vi "F6_1.vi"(8 "error in (no error)":errorcluster, 9 "data":u8[](array[numeric]), 10 "function":u8, 11 "device data model in":refnum<class "Standard Data Model1.lvclass">) -> (0 "error out":errorcluster, 1 "data return":u8[](array[numeric]), 2 "function return":u8, 3 "device data model out":refnum<class "Standard Data Model1.lvclass">)   [LabVIEW 2021, in "NI_modbus_upd.lvlib" / "Standard Data Model1.lvclass"]
doc: "Executes function code 6"
uses:
  Standard Data Model1.lvclass
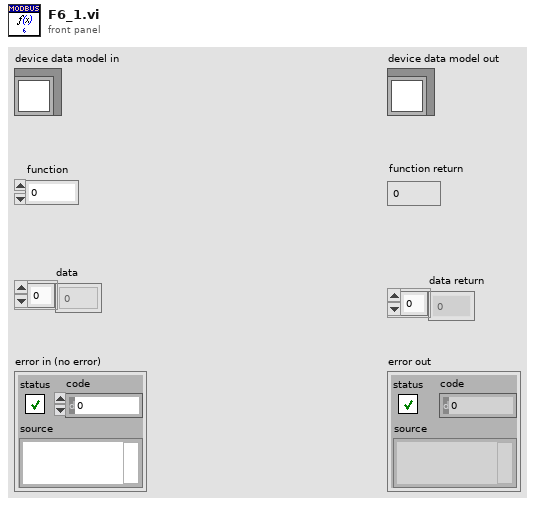
[diagram p1: front panel]
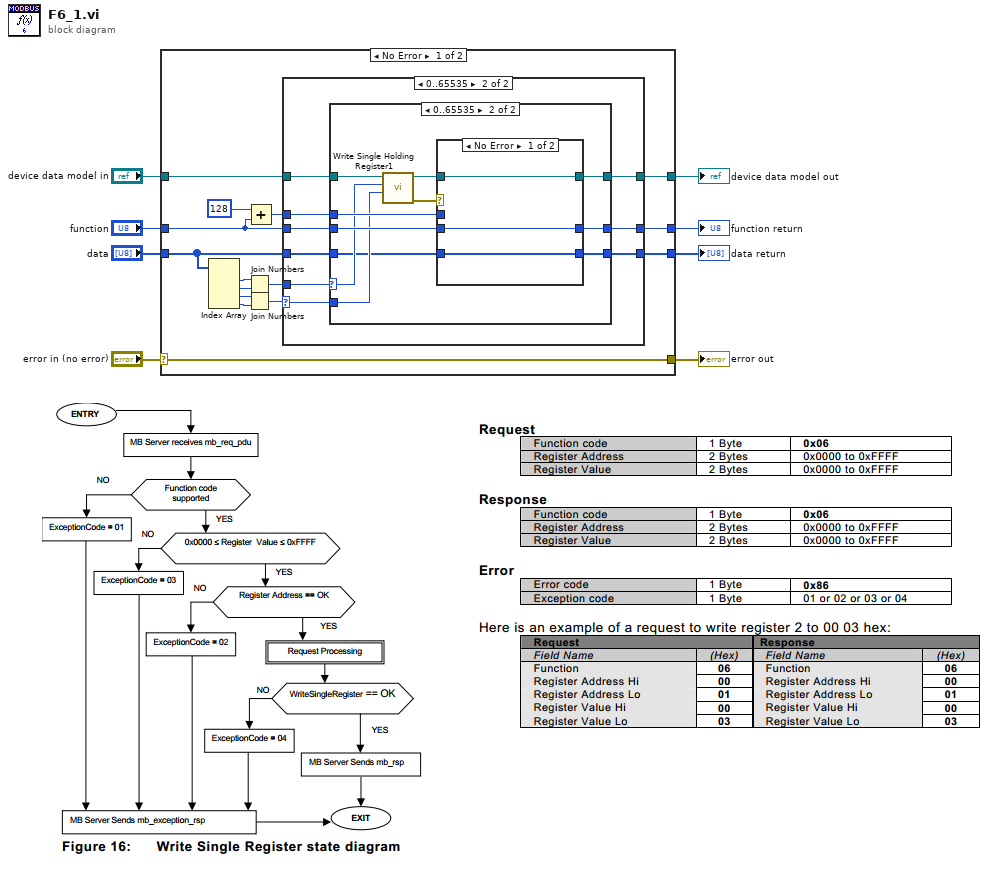
[diagram p0: block diagram]
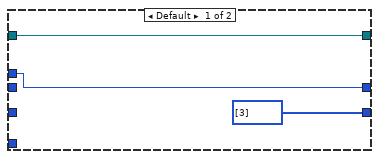
[diagram p2: hidden frame]
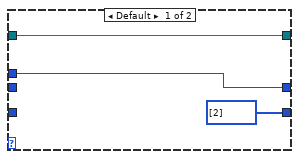
[diagram p3: hidden frame]
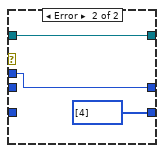
[diagram p4: hidden frame]
diagram:
  n1 = case shown="No Error" "error in (no error)" {
    selector: "error in (no error)" -> [w23 w59]
    tunnel: [w23 w59] -> w7
    tunnel: [w17 w58] -> w5
    tunnel: "device data model in" -> [w16 w58]
    tunnel: "function" -> [w13 w57]
    tunnel: "data" -> [w9 w56]
    tunnel: [w12 w57] -> w2
    tunnel: [w11 w56] -> w1
    frame No Error {
      n2 = Index Array(array=w9) -> (element #1=w21:u8, element #2=w22:u8, element #3=w20:u8, element #4=w19:u8)  [unwired: 4 in]
      n3 = Join Numbers(hi=w21, lo=w22) -> ((hi.lo)=w10:u16)
      n4 = Join Numbers(hi=w20, lo=w19) -> ((hi.lo)=w18:u16)
      n5 = Add(x=u8 128, y=w13) -> (x+y=w14:u8)
      n6 = case shown="0..65535" w18 {
        selector: w18 -> [_ w35]
        tunnel: [w26 w34] -> w17
        tunnel: w16 -> [w26 w33]
        tunnel: w14 -> [w25 w32]
        tunnel: w13 -> [_ w30]
        tunnel: [w25 w31] -> w12
        tunnel: [u8[] [3] ("Data Return") w29] -> w11
        tunnel: w10 -> [_ w28]
        tunnel: w9 -> [_ w27]
        frame Default {
        }
        frame 0..65535 {
          n7 = case shown="0..65535" w28 {
            selector: w28 -> [_ w42]
            tunnel: w35 -> [_ w43]
            tunnel: [w38 w49] -> w34
            tunnel: w33 -> [w38 w41]
            tunnel: w32 -> [w37 w48]
            tunnel: [w37 w46] -> w31
            tunnel: w30 -> [_ w47]
            tunnel: [u8[] [2] ("Data Return") w45] -> w29
            tunnel: w27 -> [_ w39]
            frame Default {
            }
            frame 0..65535 {
              n8 = call "Write Single Holding Register1.vi"("register value"=w43, "address"=w42, "device data model in"=w41) -> ("error out"=w40:errorcluster, "device data model out"=w44:refnum<class "Standard Data Model1.lvclass">)  [unwired: 7 in]
              n9 = case shown="No Error" w40 {
                tunnel: w44 -> [w52 w55]
                tunnel: [w52 w55] -> w49
                tunnel: w48 -> [_ w54]
                tunnel: w47 -> [w51 _]
                tunnel: [w51 w54] -> w46
                tunnel: [w50 u8[] [4]] -> w45
                tunnel: w39 -> [w50 _]
                frame No Error {
                }
                frame Error {
                }
              }
            }
          }
        }
      }
    }
    frame Error {
    }
  }
  "error out" <- w7
  "device data model out" <- w5
  "data return" <- w1
  "function return" <- w2
